vi "Modulator.vi"(8 "error in (no error)":errorcluster, 11 "Felica DOWN in":refnum<class "Felica DOWN.lvclass">) -> (0 "error out":errorcluster, 2 "Waveform out":waveform(dbl), 3 "Felica DOWN out":refnum<class "Felica DOWN.lvclass">)   [LabVIEW 2019, in "Felica DOWN.lvclass"]
uses:
  Felica DOWN.lvclass
  TypeDef/Store.ctl
  Felica DOWN.lvclass/Felica DOWN.ctl
  <vilib>/addons/Modulation/Analog/MT Modulate AM (DSB).vi
  <vilib>/addons/Modulation/Analog/MT Upconvert Baseband (Real).vi
  <vilib>/addons/Modulation/niAMT.lvlib
  RFID system.lvclass
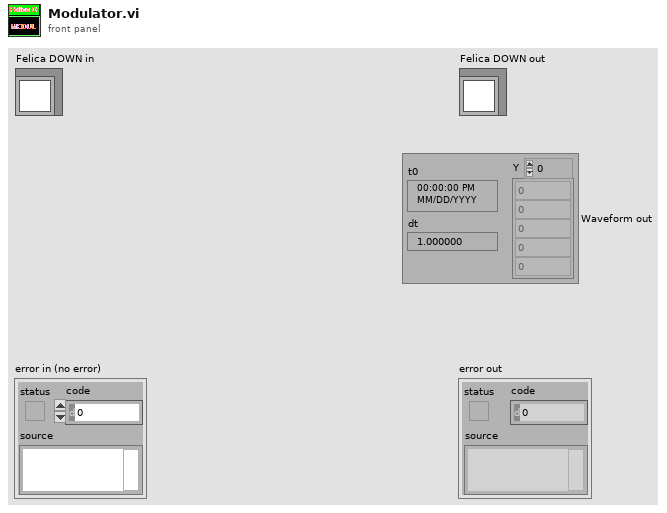
[diagram p1: front panel]
types:
  T1 = typedef "Store.ctl" = enum16{"envelope", "noise", "demSubCar", "CH_frame", "Decode", "demodulate", "in", "out", "sum", "subCarrier", "frame", "command", "encode", "modulate", "encode_UP", "modulate_up", "demod_up", "envelop_up", "sum_up", "out_up", "in_up"}
  T2 = typedef "niAMT.lvlib/Complex Data Waveform.ctl" = cluster{"t0":dbl, "dt":dbl, "Y":cdb[]}
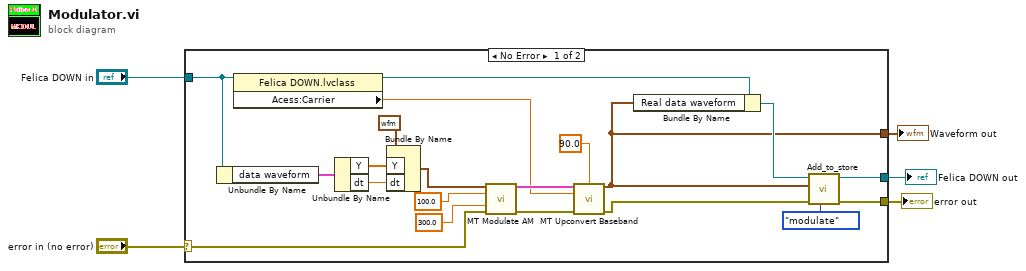
[diagram p0: block diagram]
diagram:
  n1 = case shown="No Error" "error in (no error)" {
    selector: "error in (no error)" -> [w10 w26]
    tunnel: "Felica DOWN in" -> [w16 w27]
    tunnel: [w11 w27] -> w3
    tunnel: [w8 w26] -> w2
    tunnel: [w6 _] -> w1
    frame No Error {
      n2 = Unbundle By Name(w16) -> ("data waveform"=w15:T2)
      n3 = property class="Felica DOWN.lvclass"(reference=w16) -> (reference out=w13:refnum<class "Felica DOWN.lvclass">, "Acess:Carrier"=w14:dbl)  [unwired: 1 in, 1 out]
      n4 = Unbundle By Name(w15) -> ("Y"=w22:cdb[], "dt"=w23:dbl)
      n5 = Bundle By Name(cluster=waveform(cdb) {"t0"=timestamp(0 s since 1904-01-01), "dt"=1.0, "Y"=[]} ("waveform"), "Y"=w22, "dt"=w23) -> (w20:waveform(cdb))
      n6 = call-poly <vilib>:"MT Modulate AM.vi"("message signal"=w20, "modulation index"=100.0, "peak message amplitude"=300.0, "error in (no error)"=w10) -> ("AM modulated waveform"=w21:cluster{"t0":dbl, "dt":dbl, "Y":cdb[]}, "error out"=w18:errorcluster)  [unwired: 10 in]
      n7 = call-poly <vilib>:"MT Upconvert Baseband.vi"("baseband waveform (complex)"=w21, "initial phase (deg)"=90.0, "carrier frequency (Hz)"=w14, "error in (no error)"=w18) -> ("passband waveform"=w6:waveform(dbl), "error out"=w9:errorcluster)  [unwired: 10 in]
      n8 = Bundle By Name(cluster=w13, "Real data waveform"=w6) -> (w12:refnum<class "Felica DOWN.lvclass">)
      n9 = call "Add_to_store.vi"("Store"=Store."modulate", "error in (no error)"=w9, "Waveform"=w6, "RFID system in"=w12) -> ("error out"=w8:errorcluster, "RFID system out"=w11:refnum<class "Felica DOWN.lvclass">)  [unwired: 6 in]
    }
    frame Error {
    }
  }
  "error out" <- w2
  "Felica DOWN out" <- w3
  "Waveform out" <- w1
